vi "LV Timestamp to PCAP ts.vi"(11 "LabVIEW Time Stamp":timestamp) -> (2 "ts_usec":u32, 3 "ts_sec":u32)   [LabVIEW 2025, in "Automotive Ethernet Bus Monitor UI.lvlib" / "lvwpcap.lvlib"]
uses:
  lvwpcap.lvlib
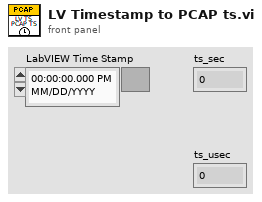
[diagram p1: front panel]
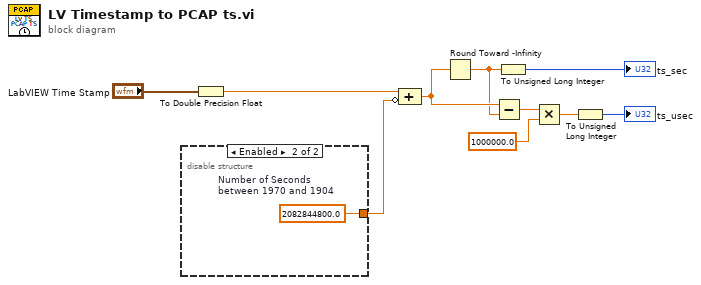
[diagram p0: block diagram]
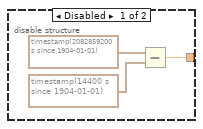
[diagram p2: hidden frame]
diagram:
  n1 = disable-structure "Diagram Disable Structure" shown="Enabled" {
    disable-tunnel: [w11 w14] -> w10
    frame Disabled {
      n2 = Subtract(x=timestamp(2082859200 s since 1904-01-01), y=timestamp(14400 s since 1904-01-01)) -> (x-y=w11:dbl)
    }
    frame Enabled {
      w14 = 2082844800.0  # Number of Seconds between 1970 and 1904
    }
  }
  n3 = To Double Precision Float(number="LabVIEW Time Stamp") -> (double precision float=w8:dbl)
  n4 = Compound Arithmetic op=ADD(w8, invert w10) -> (w6:dbl)
  n5 = Round Toward -Infinity(1:w6) -> (0:w5:dbl)
  n6 = Subtract(x=w6, y=w5) -> (x-y=w4:dbl)
  n7 = To Unsigned Long Integer(number=w5) -> (unsigned 32bit integer=→"ts_sec":u32)
  n8 = Multiply(x=w4, y=1000000.0) -> (x*y=w2:dbl)
  n9 = To Unsigned Long Integer(number=w2) -> (unsigned 32bit integer=→"ts_usec":u32)
